vi "Write Function.lvclass.vi"(10 "Function Actor.lvlib:Function.lvclass":refnum<class "Function.lvclass">, 11 "Add Available Function Msg in":refnum<class "Add Available Function Msg.lvclass">) -> (3 "Add Available Function Msg out":refnum<class "Add Available Function Msg.lvclass">)   [LabVIEW 2016, in "Controller Actor.lvlib" / "Add Available Function Msg.lvclass"]
uses:
  <userlib>/Common Components/Controller/Messages/Add Available Function Msg/Add Available Function Msg.lvclass
  <userlib>/Common Components/Function Actor/Function.lvclass
  <userlib>/Common Components/Controller/Messages/Add Available Function Msg/Add Available Function Msg.lvclass/Add Available Function Msg.ctl
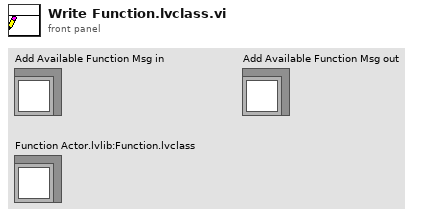
[diagram p1: front panel]
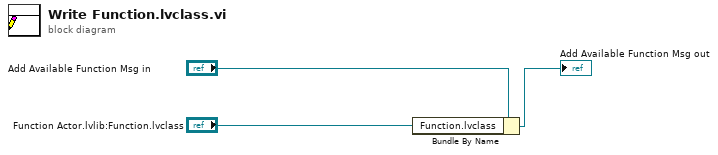
[diagram p0: block diagram]
diagram:
  n1 = Bundle By Name(cluster="Add Available Function Msg in", "Function.lvclass"="Function Actor.lvlib:Function.lvclass") -> (→"Add Available Function Msg out":refnum<class "Add Available Function Msg.lvclass">)
